vi "+S2C_Process.vi"(8 "Error In":errorcluster) -> (0 "Error Out":errorcluster)   [LabVIEW 2015]
uses:
  LVIS/Sub VIs/Globals/LVIS_DcGlobals.vi
panel:
  in  "Exit?":bool
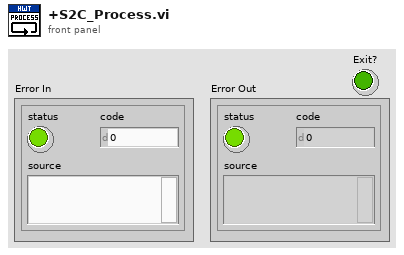
[diagram p1: front panel]
types:
  T1 = cluster{"Caller-Q":refnum<queue>, "Command":string, "Return":string, "Data":variant, "Timeout":dbl}
  T2 = enum32{"Bad", "Idle", "Run top level", "Running"}
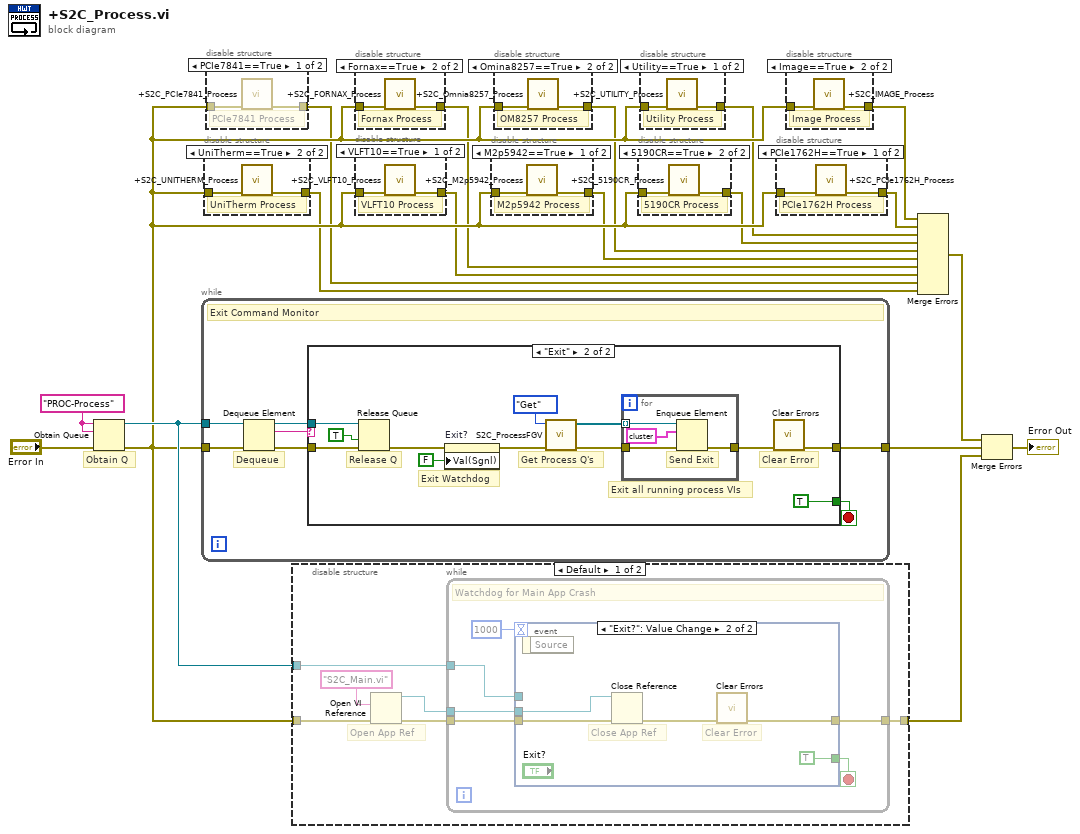
[diagram p0: block diagram]
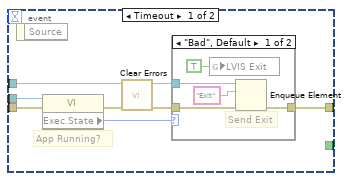
[diagram p5: hidden frame]
diagram:
  w18 = "PROC-Process" ("name (unnamed)")
  # "Obtain Q"
  n1 = Obtain Queue(name (unnamed)=w18, element data type=w18, error in (no error)="Error In") -> (queue out=w15:refnum<queue>, error out=w11:errorcluster)  [unwired: 2 in, 1 out]
  n2 = while {
    tunnel: w11 -> [w25]
    tunnel: w15 -> [w24]
    tunnel: [w21] -> w16
    stop <- w20 stop-if-true
    # "Dequeue"
    # "Exit Command Monitor"
    n3 = Dequeue Element(queue=w24, error in (no error)=w25) -> (queue out=w19:refnum<queue>, element=w22:string, error out=w23:errorcluster)  [unwired: 1 in, 1 out]
    n4 = case shown="\"Exit\"" w22 {
      tunnel: w23 -> [w26 w33]
      tunnel: [w26 w27] -> w21
      tunnel: [_ TRUE] -> w20
      tunnel: w19 -> [_ w32]
      frame "Other", Default {
      }
      frame "Exit" {
        # "Clear Error"
        # "Exit Watchdog"
        # "Release Q"
        # "Exit all running process VIs"
        # "Get Process Q's"
        n5 = Release Queue(queue=w32, force destroy? (F)=TRUE, error in (no error)=w33) -> (error out=w30:errorcluster)  [unwired: 2 out]
        n6 = property on="Exit?" class="Bool (strict)"(error in=w30, "Val(Sgnl)"=FALSE ("Value (Signaling)")) -> (error out=w29:errorcluster)  [unwired: 1 in, 1 out]
        n7 = call "S2C_ProcessFGV.vi"("Error In"=w29, "Action"=enum16{"Init", "Add", "Get"}."Get") -> ("Error Out"=w35:errorcluster, "Q-Array"=w34:refnum<queue>[])  [unwired: 8 in]
        n8 = for {
          tunnel: [w39] -> w38
          tunnel: w35 -> [w42]
          tunnel: w34 -> [w41] mode=indexing
          # "Send Exit"
          n9 = Enqueue Element(queue=w41, element=T1 {"Caller-Q"=refnum, "Command"="Exit", "Return"="", "Data"=variant, "Timeout"=0.0} ("Command Cluster"), error in (no error)=w42) -> (error out=w39:errorcluster)  [unwired: 1 in, 2 out]
        }
        n10 = call <vilib>:"Clear Errors.vi"("error in (no error)"=w38) -> ("error out"=w27:errorcluster)  [unwired: 5 in, 1 out]
      }
    }
  }
  n11 = disable-structure shown="UniTherm==True" {
    disable-tunnel: [w43 w45] -> w10
    disable-tunnel: w11 -> [w43 w44]
    frame condition #0 {
    }
    frame condition #1 (active) {
      # "UniTherm Process"
      n12 = call "+S2C_UNITHERM_Process.vi"("Error In"=w44) -> ("Error Out"=w45:errorcluster)  [unwired: 10 in]
    }
  }
  n13 = disable-structure shown="PCIe7841==True" {
    disable-tunnel: w11 -> [w47 w48]
    disable-tunnel: [w46 w48] -> w9
    frame condition #0 {
      # "PCIe7841 Process"
      n14 = call "+S2C_PCIe7841_Process.vi"("Error In"=w47) -> ("Error Out"=w46:errorcluster)  [unwired: 10 in]
    }
    frame condition #1 (active) {
    }
  }
  n15 = disable-structure shown="Default" {
    disable-tunnel: w15 -> [w54 _]
    disable-tunnel: [w53 w79] -> w14
    disable-tunnel: w11 -> [w52 w79]
    frame condition #0 {
      # "Open App Ref"
      n16 = Open VI Reference(vi path="S2C_Main.vi", error in (no error)=w52) -> (vi reference=w49:refnum<vi>, error out=w50:errorcluster)  [unwired: 4 in]
      n17 = while {
        tunnel: w50 -> [w60]
        tunnel: w49 -> [w59]
        tunnel: w54 -> [w57]
        tunnel: [w56] -> w53
        stop <- w55 stop-if-true
        # "Watchdog for Main App Crash"
        n18 = event shown="[1] \"Exit?\": Value Change" {
          selector: _ -> [_ _]
          dyn-events: _ -> [_ _]
          timeout: 1000 -> [_ _]
          tunnel: w60 -> [w67 w77]
          tunnel: w59 -> [w66 w76]
          tunnel: w57 -> [w63 _]
          tunnel: [w62 w74] -> w56
          tunnel: [_ TRUE] -> w55
          event Timeout {
            # "App Running?"
            n19 = event-data() -> ()  [unwired: 1 in, 1 out]
            n20 = property class="VI"(reference=w66, error in=w67) -> (error out=w65:errorcluster, "Exec.State"=w64:T2)  [unwired: 1 out]
            n21 = call <vilib>:"Clear Errors.vi"("error in (no error)"=w65) -> ("error out"=w61:errorcluster)  [unwired: 5 in, 1 out]
            n22 = case shown="\"Bad\", Default" w64 {
              tunnel: w61 -> [w72 w73]
              tunnel: w63 -> [w71 _]
              tunnel: [w70 w73] -> w62
              frame "Bad", Default {
                # "Send Exit"
                n23 = global write "LVIS_DcGlobals.vi" "LVIS Exit"(TRUE ("LVIS Exit")) -> ()
                n24 = Enqueue Element(queue=w71, element="Exit", error in (no error)=w72) -> (error out=w70:errorcluster)  [unwired: 1 in, 2 out]
              }
              frame "Run top level" {
                # "All good here"
              }
            }
          }
          event "Exit?": Value Change {
            # "Clear Error"
            # "Close App Ref"
            n25 = event-data() -> ()  [unwired: 1 in, 1 out]
            n26 = Close Reference(reference=w76, error in (no error)=w77) -> (error out=w75:errorcluster)
            n27 = call <vilib>:"Clear Errors.vi"("error in (no error)"=w75) -> ("error out"=w74:errorcluster)  [unwired: 5 in, 1 out]
          }
        }
      }
    }
    frame condition #1 (active) {
    }
  }
  n28 = disable-structure shown="Fornax==True" {
    disable-tunnel: [w80 w82] -> w7
    disable-tunnel: w11 -> [w80 w81]
    frame condition #0 {
    }
    frame condition #1 (active) {
      # "Fornax Process"
      n29 = call "+S2C_FORNAX_Process.vi"("Error In"=w81) -> ("Error Out"=w82:errorcluster)  [unwired: 10 in]
    }
  }
  n30 = disable-structure shown="VLFT10==True" {
    disable-tunnel: w11 -> [w84 w85]
    disable-tunnel: [w83 w85] -> w8
    frame condition #0 (active) {
      # "VLFT10 Process"
      n31 = call "+S2C_VLFT10_Process.vi"("Error In"=w84) -> ("Error Out"=w83:errorcluster)  [unwired: 10 in]
    }
    frame condition #1 {
    }
  }
  n32 = disable-structure shown="M2p5942==True" {
    disable-tunnel: w11 -> [w87 w88]
    disable-tunnel: [w86 w88] -> w6
    frame condition #0 (active) {
      # "M2p5942 Process"
      n33 = call "+S2C_M2p5942_Process.vi"("Error In"=w87) -> ("Error Out"=w86:errorcluster)  [unwired: 10 in]
    }
    frame condition #1 {
    }
  }
  n34 = disable-structure shown="Omina8257==True" {
    disable-tunnel: w11 -> [w89 w91]
    disable-tunnel: [w89 w90] -> w5
    frame condition #0 {
    }
    frame condition #1 (active) {
      # "OM8257 Process"
      n35 = call "+S2C_Omnia8257_Process.vi"("Error In"=w91) -> ("Error Out"=w90:errorcluster)  [unwired: 10 in]
    }
  }
  n36 = disable-structure shown="5190CR==True" {
    disable-tunnel: [w92 w94] -> w4
    disable-tunnel: w11 -> [w92 w93]
    frame condition #0 {
    }
    frame condition #1 (active) {
      # "5190CR Process"
      n37 = call "+S2C_5190CR_Process.vi"("Error In"=w93) -> ("Error Out"=w94:errorcluster)  [unwired: 10 in]
    }
  }
  n38 = disable-structure shown="Utility==True" {
    disable-tunnel: w11 -> [w96 w97]
    disable-tunnel: [w95 w97] -> w3
    frame condition #0 (active) {
      # "Utility Process"
      n39 = call "+S2C_UTILITY_Process.vi"("Error In"=w96) -> ("Error Out"=w95:errorcluster)  [unwired: 10 in]
    }
    frame condition #1 {
    }
  }
  n40 = disable-structure shown="PCIe1762H==True" {
    disable-tunnel: w11 -> [w99 w100]
    disable-tunnel: [w98 w100] -> w2
    frame condition #0 (active) {
      # "PCIe1762H Process"
      n41 = call "+S2C_PCIe1762H_Process.vi"("Error In"=w99) -> ("Error Out"=w98:errorcluster)  [unwired: 10 in]
    }
    frame condition #1 {
    }
  }
  n42 = disable-structure shown="Image==True" {
    disable-tunnel: [w101 w103] -> w1
    disable-tunnel: w11 -> [w101 w102]
    frame condition #0 {
    }
    frame condition #1 (active) {
      # "Image Process"
      n43 = call "+S2C_IMAGE_Process.vi"("Error In"=w102) -> ("Error Out"=w103:errorcluster)  [unwired: 10 in]
    }
  }
  n44 = Merge Errors(w1, w2, w3, w4, w5, w6, w7, w8, w9, w10) -> (w12:errorcluster)
  n45 = Merge Errors(w12, w16, w14) -> (→"Error Out":errorcluster)
